vi "Operaciones con Strings.vi"() -> ()   [LabVIEW 2022 SP3]
panel:
  out "decimal integer string":string
  out "Thermometer 3":dbl(slide) scale=0.0..100.0
  out "Thermometer 2":dbl(slide) scale=0.0..100.0 scale format="%#_6f"
  in  "PWM 0-100%":dbl(knob) scale=0.0..100.0
  out "Thermometer":dbl(slide) scale=0.0..100.0
  out "TERCER DATO 3":string
  out "SEGUNDO DATO 2":string
  out "PRIMER DATO 2":string
  in  "Datos Rx HARDWARE 2":string
  out "Palabra invertida":string
  out "first char last":string
  out "TEXTO RESULTADO 3":string caption="Result"
  out "TEXTO RESULTADO 2":string caption="Result"
  in  "TEXTO INICIAL 2":string caption="Beginning Text"
  in  "TEXTO INICIAL":string caption="Beginning Text"
  out "TEXTO RESULTADO":string caption="Result"
  out "RESIDUO":string
  out "match substring":string
  out "SGUNDO DATO":string
  out "RESIDUO":string
  out "CARACTER SEPARADOR":string
  out "PRIMER DATO":string
  in  "Datos Rx HARDWARE":string
  out "Palabra buscada y remplazada":string
  out "Palabra Remplazada":string
  out "Remplazo de string":string
  in  "tamaño del texto":i32
  in  "offset (0)":i32
  out "Extraccion de string":string
  out "TAMAÑO 2 PALABRA CONCATENADA":i32
  out "INDICADOR CONCATENADO":string
  in  "CONTROL STRING 2":string
  out "TAMAÑO":i32
  out "INDICADOR":string
  in  "CONTROL STRING":string
  # "Teoria"
  # "Ejercicios"
  # "Ejemplo 1: DATO ADQUIRIDO"
  # "SENSOR1,SENSOR2,SENSOR3F : 50.32,45.334,12.879F"
  # "BUILT TEXT  EXPRESS VI"
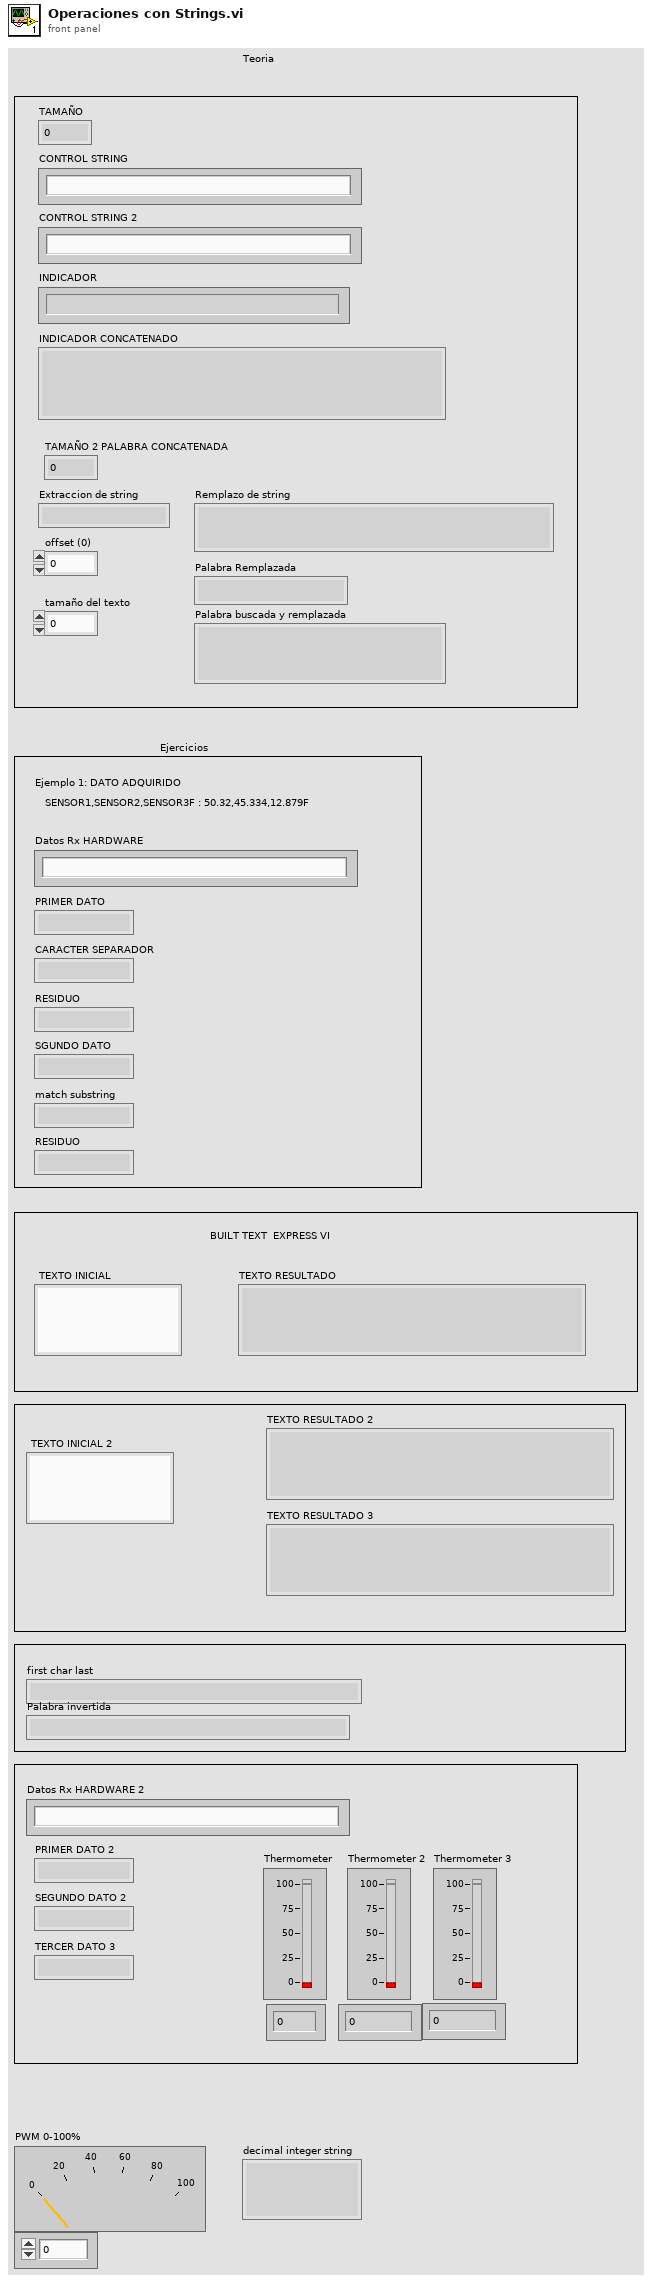
[diagram p1: front panel]
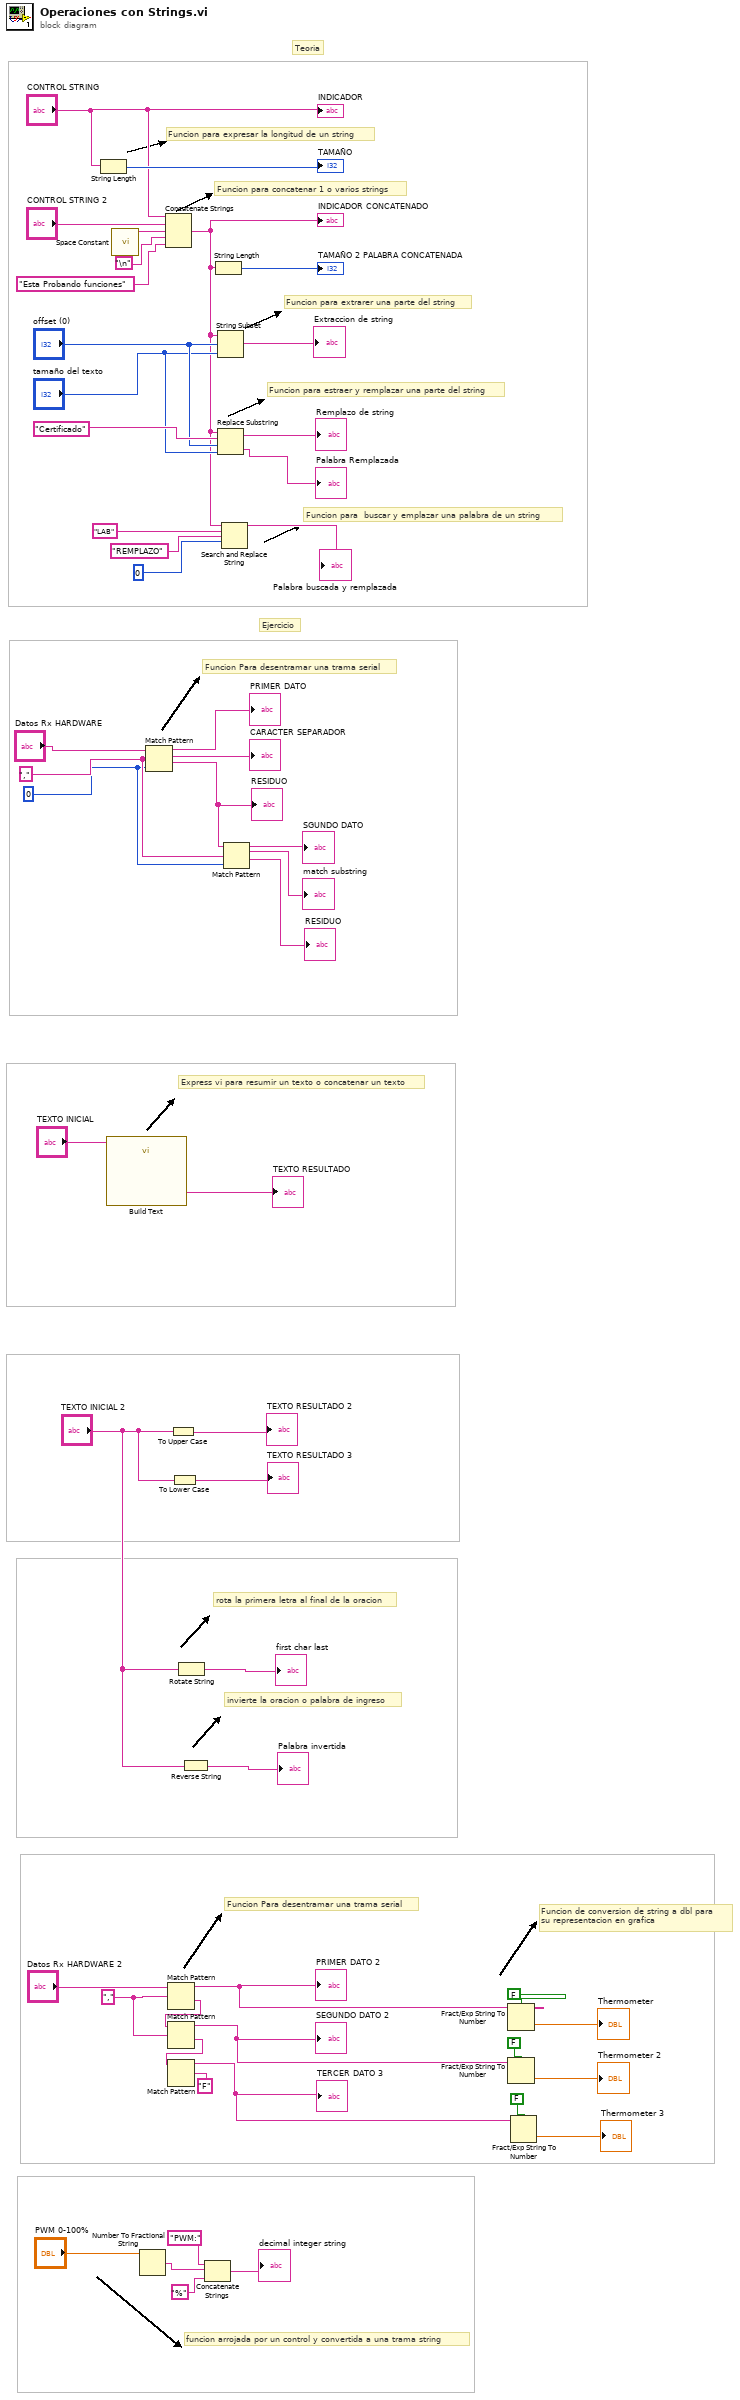
[diagram p0: block diagram]
diagram:
  w8 = "," ("regular expression")
  w30 = 0 ("offset (0)")
  w31 = "," ("regular expression")
  # "funcion arrojada por un control y convertida a una trama string"
  # "Funcion de conversion de string a dbl para\nsu representacion en grafica"
  # "Funcion Para desentramar una trama serial"
  # "invierte la oracion o palabra de ingreso"
  # "rota la primera letra al final de la oracion"
  # "Express vi para resumir un texto o concatenar un texto"
  # "Funcion Para desentramar una trama serial"
  # "Ejercicio"
  # "Teoria"
  # "Funcion para  buscar y emplazar una palabra de un string"
  # "Funcion para estraer y remplazar una parte del string"
  # "Funcion para extrarer una parte del string"
  # "Funcion para concatenar 1 o varios strings"
  # "Funcion para expresar la longitud de un string"
  n1 = String Length(string="CONTROL STRING") -> (length=→"TAMAÑO":i32)
  n2 = call "Build Text"("Beginning Text"="TEXTO INICIAL") -> ("Result"=→"TEXTO RESULTADO":string)  [unwired: 13 in, 1 out]
  n3 = call <vilib>:"Space Constant.vi"() -> ("String"=w49:string)
  n4 = Number To Fractional String(number="PWM 0-100%") -> (F-format string=w2:string)  [unwired: 3 in]
  n5 = Match Pattern(string="Datos Rx HARDWARE", regular expression=w31, offset (0)=w30) -> (before substring=→"PRIMER DATO":string, match substring=→"CARACTER SEPARADOR":string, after substring=w32:string)  [unwired: 1 out]
  "RESIDUO" <- w32
  n6 = Concatenate Strings("CONTROL STRING", "CONTROL STRING 2", w49, "\n", "Esta Probando funciones") -> (w41:string)
  "INDICADOR CONCATENADO" <- w41
  n7 = Match Pattern(string="Datos Rx HARDWARE 2", regular expression=w8) -> (before substring=w14:string, after substring=w18:string)  [unwired: 1 in, 2 out]
  "PRIMER DATO 2" <- w14
  n8 = Match Pattern(string=w18, regular expression=w8) -> (before substring=w7:string, after substring=w11:string)  [unwired: 1 in, 2 out]
  "SEGUNDO DATO 2" <- w7
  n9 = Match Pattern(string=w11, regular expression="F") -> (before substring=w6:string)  [unwired: 1 in, 3 out]
  "TERCER DATO 3" <- w6
  n10 = To Upper Case(1:"TEXTO INICIAL 2") -> (0:→"TEXTO RESULTADO 2":string)
  n11 = To Lower Case(string="TEXTO INICIAL 2") -> (all lower case string=→"TEXTO RESULTADO 3":string)
  n12 = Rotate String(1:"TEXTO INICIAL 2") -> (0:→"first char last":string)
  n13 = Reverse String(1:"TEXTO INICIAL 2") -> (0:→"Palabra invertida":string)
  n14 = Concatenate Strings("PWM:" ("string"), w2, "%" ("string")) -> (→"decimal integer string":string)
  n15 = String Length(string=w41) -> (length=→"TAMAÑO 2 PALABRA CONCATENADA":i32)
  n16 = String Subset(string=w41, offset (0)="offset (0)", length (rest)="tamaño del texto") -> (substring=→"Extraccion de string":string)
  n17 = Replace Substring(2:"tamaño del texto", 3:"offset (0)", 4:"Certificado", 5:w41) -> (0:→"Palabra Remplazada":string, 1:→"Remplazo de string":string)
  n18 = Search and Replace String(input string=w41, search string="LAB", replace string="REMPLAZO" ("replace string (\"\")"), offset=0 ("offset (0)")) -> (result string=→"Palabra buscada y remplazada":string)  [unwired: 4 in, 3 out]
  n19 = Match Pattern(string=w32, regular expression=w31, offset (0)=w30) -> (before substring=→"SGUNDO DATO":string, match substring=→"match substring":string, after substring=→"RESIDUO":string)  [unwired: 1 out]
  n20 = Fract/Exp String To Number(use system decimal point (T)=FALSE, string=w14) -> (number=→"Thermometer":dbl)  [unwired: 2 in, 1 out]
  n21 = Fract/Exp String To Number(use system decimal point (T)=FALSE, string=w7) -> (number=→"Thermometer 2":dbl)  [unwired: 2 in, 1 out]
  n22 = Fract/Exp String To Number(use system decimal point (T)=FALSE, string=w6) -> (number=→"Thermometer 3":dbl)  [unwired: 2 in, 1 out]
  "INDICADOR" <- "CONTROL STRING"
